vi "Query Status.vi"(6 "Memory Address(0)":dbl format="%#_2g", 8 "error in (no error)":errorcluster, 9 "Mask Value(0)":dbl format="%#.2f", 10 "Command (0:*CLS)":u16(ring) items=["*CLS", "*ESE", "*ESE?", "*RST", "*SRE", "*SRE?", "*STB?", "*ESR?", "*IDN?", "*OPC", "*OPC?", "*SAV", "*RCL", "*TRG", "Output State", "Output-Timer", "Output-Timer-State", "Digital Function", "Digital Output Port- State"], 11 "VISA resource name":refnum<visa-resource-name>) -> (0 "error out":errorcluster, 2 "Instrument Response":string, 3 "VISA resource name out":refnum<visa-resource-name>)   [LabVIEW 2021, in "Keithley 2200 Series.lvlib"]
doc: "Sends IEEE 488 common commands and returns the response for queries ."
uses:
  <instrlib>/Keithley 2200 Series/Keithley 2200 Series.lvlib
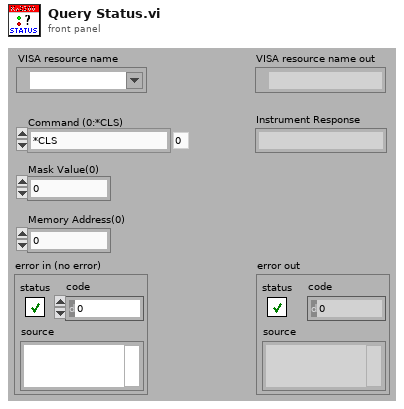
[diagram p1: front panel]
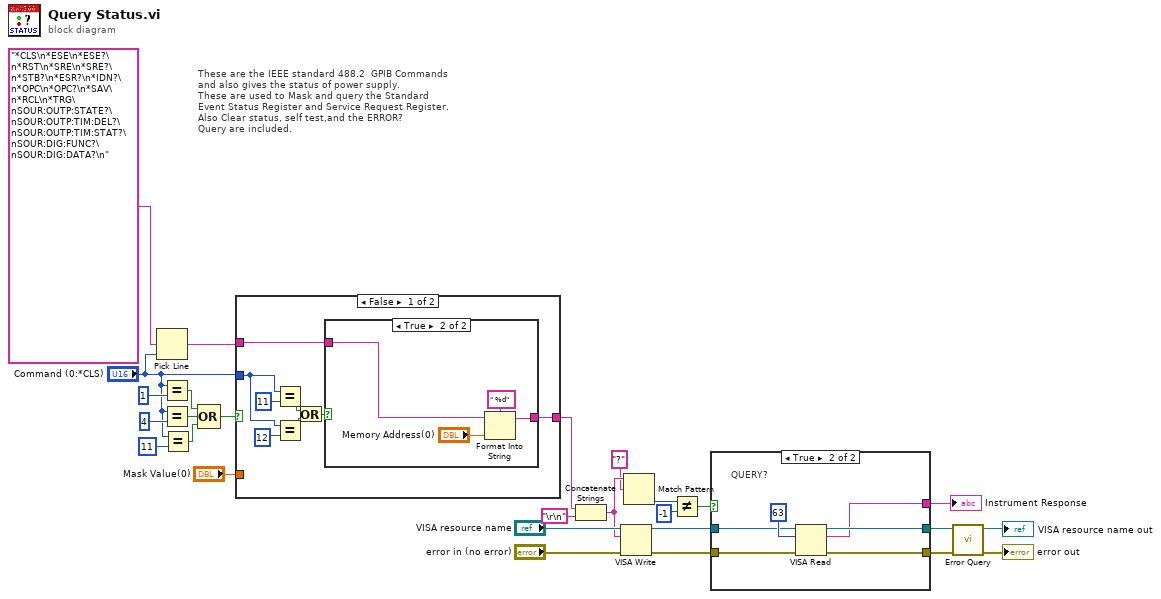
[diagram p0: block diagram]
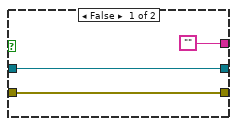
[diagram p2: hidden frame]
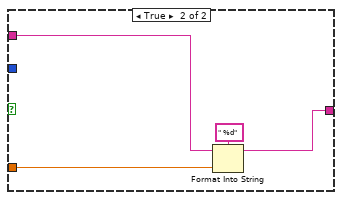
[diagram p4: hidden frame]
diagram:
  # "These are the IEEE standard 488.2  GPIB Commands\nand also gives the status of power supply.\nThese are used to Mask and query the Standard \nEvent Status Register and Service Request Register.  \nAlso Clear status, self test,and the ERROR?\nQuery are included."
  n1 = Pick Line(multi-line string="*CLS\n*ESE\n*ESE?\n*RST\n*SRE\n*SRE?\n*STB?\n*ESR?\n*IDN?\n*OPC\n*OPC?\n*SAV\n*RCL\n*TRG\nSOUR:OUTP:STATE?\nSOUR:OUTP:TIM:DEL?\nSOUR:OUTP:TIM:STAT?\nSOUR:DIG:FUNC?\nSOUR:DIG:DATA?\n", line index="Command (0:*CLS)") -> (output string=w24:string)  [unwired: 1 out]
  n2 = Equal?(x="Command (0:*CLS)", y=u16 1) -> (x = y?=w23:bool)
  n3 = Equal?(x="Command (0:*CLS)", y=u16 4) -> (x = y?=w22:bool)
  n4 = Equal?(x="Command (0:*CLS)", y=u16 11) -> (x = y?=w1:bool)
  n5 = Compound Arithmetic op=OR(w23, w22, w1) -> (w19:bool)
  n6 = case shown="False" w19 {
    tunnel: w24 -> [w35 w43]
    tunnel: [w34 w42] -> w11
    tunnel: "Mask Value(0)" -> [_ w41]
    tunnel: "Command (0:*CLS)" -> [w28 _]
    frame False {
      n7 = Equal?(x=w28, y=u16 11) -> (x = y?=w30:bool)
      n8 = Equal?(x=w28, y=u16 12) -> (x = y?=w29:bool)
      n9 = Or(x=w30, y=w29) -> (x .or. y?=w31:bool)
      n10 = case shown="True" w31 {
        tunnel: w35 -> [w36 w39]
        tunnel: [w36 w38] -> w34
        frame False {
        }
        frame True {
          n11 = Format Into String(format string=" %d", initial string=w39, "Memory Address(0)") -> (resulting string=w38:string)  [unwired: 1 in, 1 out]
        }
      }
    }
    frame True {
      n12 = Format Into String(format string=" %d", initial string=w43, w41) -> (resulting string=w42:string)  [unwired: 1 in, 1 out]
    }
  }
  n13 = Concatenate Strings(w11, "\r\n" ("End of Line Constant")) -> (w10:string)
  n14 = VISA Write(VISA resource name="VISA resource name", write buffer=w10, error in (no error)="error in (no error)") -> (VISA resource name out=w16:refnum<visa-resource-name>, error out=w18:errorcluster)  [unwired: 1 out]
  n15 = Match Pattern(string=w10, regular expression="?") -> (offset past match=w25:i32)  [unwired: 4 out]
  n16 = Not Equal?(x=w25, y=-1) -> (x != y?=w17:bool)
  n17 = case shown="True" w17 {
    tunnel: [w47 w53] -> w6
    tunnel: w18 -> [w47 w52]
    tunnel: w16 -> [w46 w50]
    tunnel: [w46 w49] -> w7
    tunnel: ["" ("read buffer") w48] -> w12
    frame False {
    }
    frame True {
      # "QUERY?"
      n18 = VISA Read(VISA resource name=w50, byte count=u32 63, error in (no error)=w52) -> (VISA resource name out=w49:refnum<visa-resource-name>, read buffer=w48:string, error out=w53:errorcluster)  [unwired: 1 out]
    }
  }
  "Instrument Response" <- w12
  n19 = call <instrlib>:"Error Query.vi"("error in (no error)"=w6, "VISA resource name"=w7) -> ("error out"=→"error out":errorcluster, "VISA resource name out"=→"VISA resource name out":refnum<visa-resource-name>)  [unwired: 8 out]
